vi "Read TestComplete Infomation.vi"(7 "timeout ms (-1)":i32=-1, 8 "error in (no error)":errorcluster, 11 "endpoint in":refnum<k21>) -> (0 "error out":errorcluster, 1 "SerialNumber":string, 2 "Test Result":bool, 3 "endpoint out":refnum<k21>, 4 "Socket":i32)   [LabVIEW 2019, in "Test Bench Tools.lvlib"]
uses:
  Test Bench Tools.lvlib
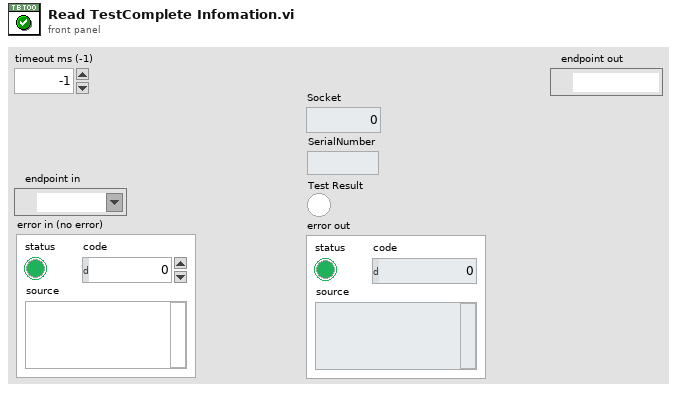
[diagram p1: front panel]
types:
  T1 = cluster{"Socket":i32, "SerialNumber":string, "TestResult":string}
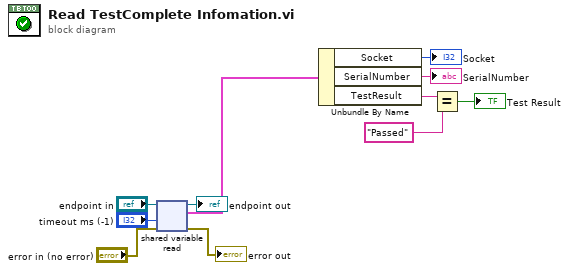
[diagram p0: block diagram]
diagram:
  n1 = shared-variable-read("endpoint in", "error in (no error)", "timeout ms (-1)") -> (→"endpoint out":refnum<k21>, →"error out":errorcluster, w8:T1)  [unwired: 1 out]
  n2 = Unbundle By Name(w8) -> ("Socket"=→"Socket":i32, "SerialNumber"=→"SerialNumber":string, "TestResult"=w5:string)
  n3 = Equal?(x=w5, y="Passed") -> (x = y?=→"Test Result":bool)
